vi "K-Mean Clustering.vi"() -> ()   [LabVIEW 2017]
uses:
  <vilib>/addons/Time Series Analysis/Statistical Analysis.llb/TSA Covariance (Array).vi
  <vilib>/Analysis/NI_AALBase.lvlib
  <vilib>/addons/_Advanced Signal Processing/NI_AdvSigProcTSA.lvlib
panel:
  out "Current calculated centroids means":dbl[](array[numeric])
  out "Previous  centroids means":dbl[](array[numeric])
  in  "milliseconds to wait":u32=2000
  out "i":i32
  out "Waveform Graph":dbl[](graph)
  out "mean 5":dbl format="%0.2f"
  out "variance 5":dbl format="%0.2f"
  out "mean 4":dbl format="%0.2f"
  out "variance 4":dbl format="%0.2f"
  out "mean 3":dbl format="%0.2f"
  out "variance 3":dbl format="%0.2f"
  out "mean 2":dbl format="%0.2f"
  out "variance 2":dbl format="%0.2f"
  out "min value":dbl
  out "max value":dbl
  out "appended array":dbl[](array[numeric])
  out "element":dbl
  out "DOA Gp 5":dbl[](array[numeric])
  out "DOA Gp 4":dbl[](array[numeric])
  out "DOA Gp 3":dbl[](array[numeric])
  out "DOA Gp 2":dbl[](array[numeric])
  out "Group?":i32
  out "variance":dbl format="%0.2f"
  out "mean":dbl format="%0.2f"
  out "DOA Gp 1":dbl[](array[numeric])
  in  "Data":dbl[](array[numeric])=[11.0, 12.0, 13.0, 21.0, 22.0, 23.0, 31.0, 32.0, 33.0, 41.0, 42.0, 43.0, 51.0, 52.0, 53.0]
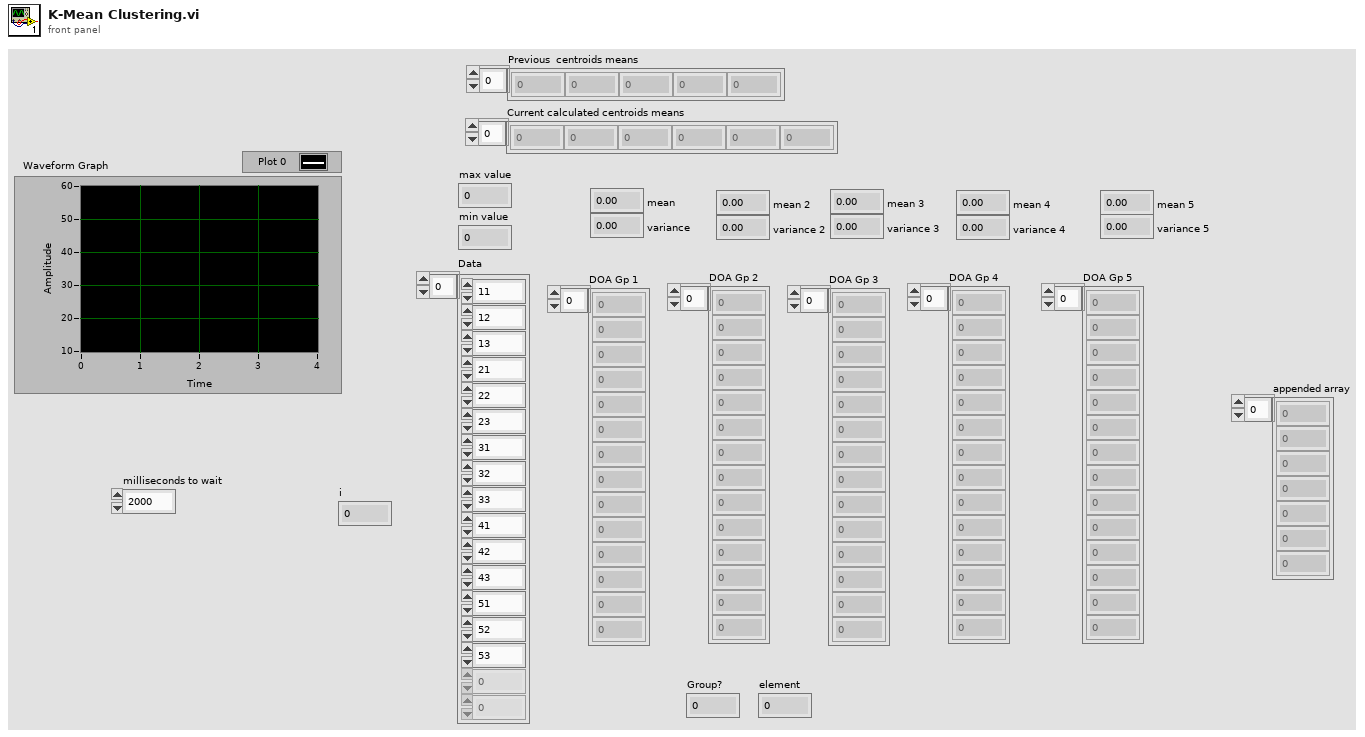
[diagram p1: front panel]
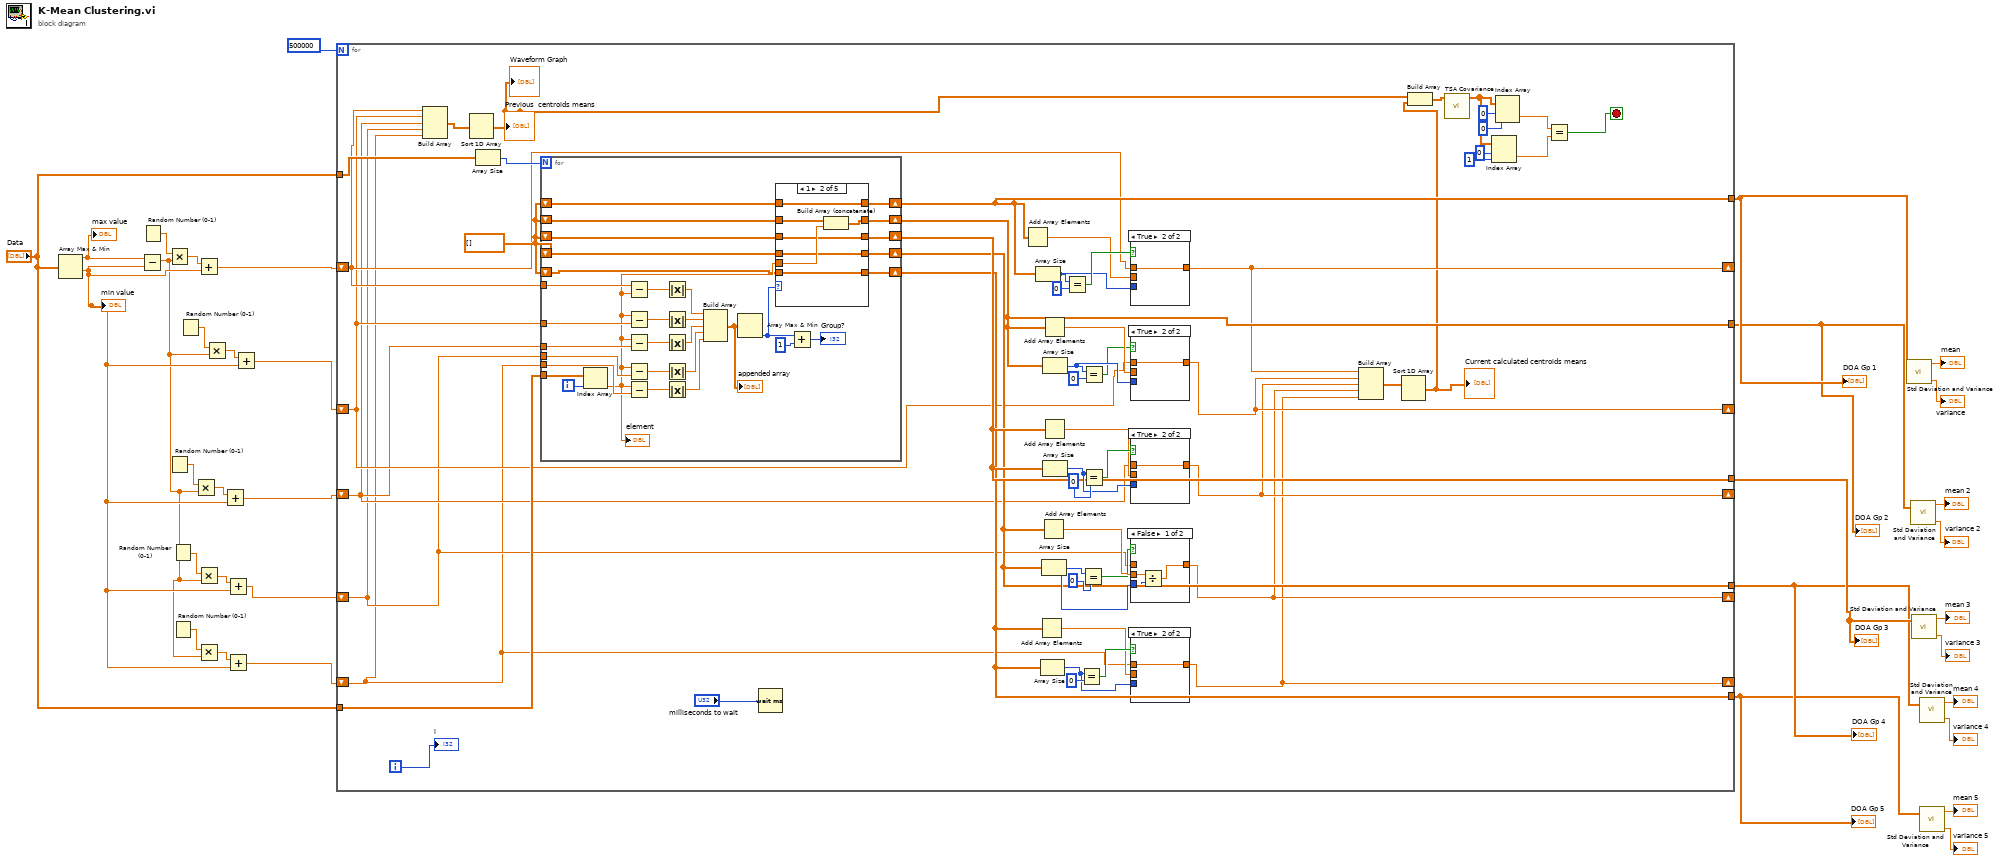
[diagram p0: block diagram]
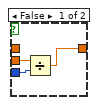
[diagram p2: hidden frame]
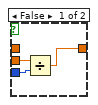
[diagram p4: hidden frame]
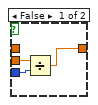
[diagram p5: hidden frame]
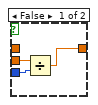
[diagram p6: hidden frame]
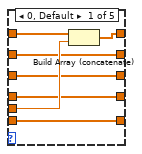
[diagram p7: hidden frame]
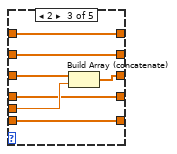
[diagram p8: hidden frame]
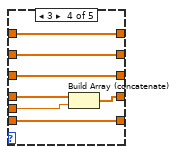
[diagram p9: hidden frame]
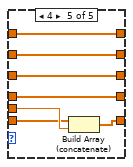
[diagram p10: hidden frame]
diagram:
  n1 = Array Max & Min(array="Data") -> (max value=w30:dbl, min value=w2:dbl)  [unwired: 2 out]
  "max value" <- w30
  "min value" <- w2
  n2 = Subtract(x=w30, y=w2) -> (x-y=w1:dbl)
  n3 = Random Number (0-1)() -> (number: 0 to 1=w17:dbl)
  n4 = Multiply(x=w17, y=w1) -> (x*y=w16:dbl)
  n5 = Random Number (0-1)() -> (number: 0 to 1=w12:dbl)
  n6 = Random Number (0-1)() -> (number: 0 to 1=w9:dbl)
  n7 = Random Number (0-1)() -> (number: 0 to 1=w6:dbl)
  n8 = Random Number (0-1)() -> (number: 0 to 1=w13:dbl)
  n9 = Multiply(x=w12, y=w1) -> (x*y=w11:dbl)
  n10 = Add(x=w16, y=w2) -> (x+y=w15:dbl)
  n11 = Multiply(x=w9, y=w1) -> (x*y=w10:dbl)
  n12 = Multiply(x=w6, y=w1) -> (x*y=w5:dbl)
  n13 = Multiply(x=w13, y=w1) -> (x*y=w14:dbl)
  n14 = Add(x=w11, y=w2) -> (x+y=w7:dbl)
  n15 = Add(x=w10, y=w2) -> (x+y=w4:dbl)
  n16 = Add(x=w5, y=w2) -> (x+y=w3:dbl)
  n17 = Add(x=w14, y=w2) -> (x+y=w8:dbl)
  n18 = for {
    N: 500000 -> [_]
    tunnel: "Data" -> [w88]
    shift-right: [w43] -> _
    shift-left: w15 -> [w57]
    shift-right: [w42] -> _
    shift-left: w8 -> [w56]
    tunnel: [w87] -> w32
    shift-right: [w41] -> _
    shift-left: w7 -> [w55]
    shift-right: [w40] -> _
    shift-left: w4 -> [w54]
    shift-right: [w39] -> _
    shift-left: w3 -> [w53]
    tunnel: "Data" -> [w85]
    tunnel: [w76] -> w27
    tunnel: [w71] -> w24
    tunnel: [w62] -> w19
    tunnel: [w61] -> w18
    i -> [w59]
    stop <- w36 stop-if-true
    w86 = dbl[] []
    n19 = Build Array(w57, w56, w55, w54, w53) -> (w58:dbl[])
    n20 = Sort 1D Array(array=w58) -> (sorted array=w44:dbl[])
    "Waveform Graph" <- w44
    "Previous  centroids means" <- w44
    n21 = Array Size(array=w85) -> (size(s)=w89:i32)
    n22 = for {
      N: w89 -> [_]
      tunnel: w88 -> [w141]
      tunnel: w57 -> [w137]
      tunnel: w56 -> [w136]
      shift-right: [w122] -> w87
      shift-left: w86 -> [w121]
      shift-right: [w120] -> w76
      shift-left: w86 -> [w119]
      tunnel: w55 -> [w129]
      tunnel: w54 -> [w128]
      tunnel: w53 -> [w127]
      shift-right: [w118] -> w71
      shift-left: w86 -> [w117]
      shift-right: [w116] -> w62
      shift-left: w86 -> [w115]
      shift-right: [w113] -> w61
      shift-left: w86 -> [w114]
      i -> [w140]
      n23 = Index Array(array=w141, index=w140) -> (element=w123:dbl)
      "element" <- w123
      n24 = Subtract(x=w137, y=w123) -> (x-y=w139:dbl)
      n25 = Subtract(x=w123, y=w136) -> (x-y=w138:dbl)
      n26 = Subtract(x=w123, y=w129) -> (x-y=w132:dbl)
      n27 = Subtract(x=w123, y=w128) -> (x-y=w131:dbl)
      n28 = Subtract(x=w123, y=w127) -> (x-y=w130:dbl)
      n29 = Absolute Value(x=w139) -> (abs(x)=w135:dbl)
      n30 = Absolute Value(x=w138) -> (abs(x)=w134:dbl)
      n31 = Absolute Value(x=w132) -> (abs(x)=w126:dbl)
      n32 = Absolute Value(x=w131) -> (abs(x)=w125:dbl)
      n33 = Absolute Value(x=w130) -> (abs(x)=w124:dbl)
      n34 = Build Array(w135, w134, w126, w125, w124) -> (w133:dbl[])
      "appended array" <- w133
      n35 = Array Max & Min(array=w133) -> (min index (indices)=w112:i32)  [unwired: 3 out]
      n36 = case shown="1" w112 {
        tunnel: w123 -> [w148 w155 w162 w169 w176]
        tunnel: [w147 w152 w159 w166 w173] -> w122
        tunnel: w121 -> [w146 w152 w159 w166 w173]
        tunnel: [w145 w154 w158 w165 w172] -> w120
        tunnel: w119 -> [w145 w153 w158 w165 w172]
        tunnel: [w144 w151 w161 w164 w171] -> w118
        tunnel: w117 -> [w144 w151 w160 w164 w171]
        tunnel: [w143 w150 w157 w168 w170] -> w116
        tunnel: w115 -> [w143 w150 w157 w167 w170]
        tunnel: w114 -> [w142 w149 w156 w163 w175]
        tunnel: [w142 w149 w156 w163 w174] -> w113
        frame 0, Default {
          n37 = Build Array (concatenate)(w146, w148) -> (w147:dbl[])
        }
        frame 1 {
          n38 = Build Array (concatenate)(w153, w155) -> (w154:dbl[])
        }
        frame 2 {
          n39 = Build Array (concatenate)(w160, w162) -> (w161:dbl[])
        }
        frame 3 {
          n40 = Build Array (concatenate)(w167, w169) -> (w168:dbl[])
        }
        frame 4 {
          n41 = Build Array (concatenate)(w175, w176) -> (w174:dbl[])
        }
      }
      n42 = Add(x=w112, y=1) -> (x+y=→"Group?":i32)
    }
    n43 = Wait (ms)(milliseconds to wait="milliseconds to wait") -> ()  [unwired: 1 out]
    n44 = Add Array Elements(numeric array=w87) -> (sum=w81:dbl)
    n45 = Array Size(array=w87) -> (size(s)=w82:i32)
    n46 = Add Array Elements(numeric array=w61) -> (sum=w63:dbl)
    n47 = Array Size(array=w61) -> (size(s)=w64:i32)
    n48 = Add Array Elements(numeric array=w62) -> (sum=w70:dbl)
    n49 = Add Array Elements(numeric array=w76) -> (sum=w80:dbl)
    n50 = Add Array Elements(numeric array=w71) -> (sum=w72:dbl)
    n51 = Array Size(array=w62) -> (size(s)=w69:i32)
    n52 = Array Size(array=w76) -> (size(s)=w79:i32)
    n53 = Array Size(array=w71) -> (size(s)=w73:i32)
    n54 = Equal?(x=w82, y=0) -> (x = y?=w83:bool)
    n55 = Equal?(x=w64, y=0) -> (x = y?=w65:bool)
    n56 = Equal?(x=w69, y=0) -> (x = y?=w68:bool)
    n57 = Equal?(x=w79, y=0) -> (x = y?=w78:bool)
    n58 = Equal?(x=w73, y=0) -> (x = y?=w74:bool)
    n59 = case shown="True" w83 {
      tunnel: [w108 w109] -> w43
      tunnel: w82 -> [w107 _]
      tunnel: w81 -> [w106 _]
      tunnel: w57 -> [_ w109]
      frame False {
        n60 = Divide(x=w106, y=w107) -> (x/y=w108:dbl)
      }
      frame True {
      }
    }
    n61 = case shown="True" w78 {
      tunnel: [w104 w105] -> w42
      tunnel: w79 -> [w103 _]
      tunnel: w80 -> [w102 _]
      tunnel: w56 -> [_ w105]
      frame False {
        n62 = Divide(x=w102, y=w103) -> (x/y=w104:dbl)
      }
      frame True {
      }
    }
    n63 = case shown="True" w74 {
      tunnel: [w100 w101] -> w41
      tunnel: w73 -> [w99 _]
      tunnel: w72 -> [w98 _]
      tunnel: w55 -> [_ w101]
      frame False {
        n64 = Divide(x=w98, y=w99) -> (x/y=w100:dbl)
      }
      frame True {
      }
    }
    n65 = case shown="False" w68 {
      tunnel: [w96 w97] -> w40
      tunnel: w69 -> [w95 _]
      tunnel: w70 -> [w94 _]
      tunnel: w54 -> [_ w97]
      frame False {
        n66 = Divide(x=w94, y=w95) -> (x/y=w96:dbl)
      }
      frame True {
      }
    }
    n67 = case shown="True" w65 {
      tunnel: [w92 w93] -> w39
      tunnel: w64 -> [w91 _]
      tunnel: w63 -> [w90 _]
      tunnel: w53 -> [_ w93]
      frame False {
        n68 = Divide(x=w90, y=w91) -> (x/y=w92:dbl)
      }
      frame True {
      }
    }
    n69 = Build Array(w43, w42, w41, w40, w39) -> (w38:dbl[])
    n70 = Sort 1D Array(array=w38) -> (sorted array=w37:dbl[])
    "Current calculated centroids means" <- w37
    n71 = Build Array(w44, w37) -> (w52:dbl[][])
    n72 = call-poly <vilib>:"TSA Covariance.vi"("Xt"=w52) -> ("covariance"=w51:dbl[][])  [unwired: 9 in, 1 out]
    n73 = Index Array(array=w51, index (row)=0, index (col)=1 ("disabled index (col)")) -> (element=w45:dbl)
    n74 = Index Array(array=w51, index (row)=0, index (col)=0 ("disabled index (col)")) -> (element=w46:dbl)
    n75 = Equal?(x=w46, y=w45) -> (x = y?=w36:bool)
    "i" <- w59
  }
  "DOA Gp 1" <- w32
  "DOA Gp 2" <- w27
  "DOA Gp 3" <- w24
  "DOA Gp 4" <- w19
  "DOA Gp 5" <- w18
  n76 = call <vilib>:"Std Deviation and Variance.vi"("X"=w32) -> ("mean"=→"mean":dbl, "variance"=→"variance":dbl)  [unwired: 1 in, 1 out]
  n77 = call <vilib>:"Std Deviation and Variance.vi"("X"=w27) -> ("mean"=→"mean 2":dbl, "variance"=→"variance 2":dbl)  [unwired: 1 in, 1 out]
  n78 = call <vilib>:"Std Deviation and Variance.vi"("X"=w24) -> ("mean"=→"mean 3":dbl, "variance"=→"variance 3":dbl)  [unwired: 1 in, 1 out]
  n79 = call <vilib>:"Std Deviation and Variance.vi"("X"=w19) -> ("mean"=→"mean 4":dbl, "variance"=→"variance 4":dbl)  [unwired: 1 in, 1 out]
  n80 = call <vilib>:"Std Deviation and Variance.vi"("X"=w18) -> ("mean"=→"mean 5":dbl, "variance"=→"variance 5":dbl)  [unwired: 1 in, 1 out]
